vi "C_F.vi"() -> ()   [LabVIEW 2014]
panel:
  in  "STOP":bool
  in  "Temp Scale":bool
  out "Thermometer":dbl(slide) scale=0.0..100.0
  # "C\n\nF"
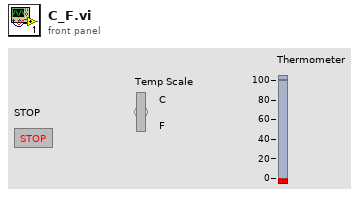
[diagram p1: front panel]
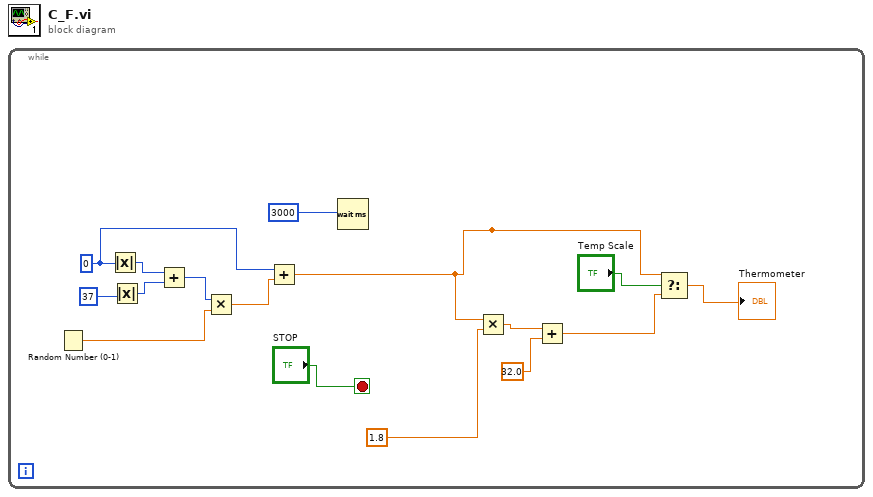
[diagram p0: block diagram]
diagram:
  n1 = while {
    stop <- "STOP" stop-if-true
    w11 = 0
    n2 = Random Number (0-1)() -> (number: 0 to 1=w13:dbl)
    n3 = Absolute Value(x=w11) -> (abs(x)=w15:i32)
    n4 = Absolute Value(x=37) -> (abs(x)=w14:i32)
    n5 = Add(x=w15, y=w14) -> (x+y=w12:i32)
    n6 = Multiply(x=w12, y=w13) -> (x*y=w10:dbl)
    n7 = Add(x=w11, y=w10) -> (x+y=w1:dbl)
    n8 = Wait (ms)(milliseconds to wait=3000) -> ()  [unwired: 1 out]
    n9 = Multiply(x=w1, y=1.8) -> (x*y=w4:dbl)
    n10 = Add(x=w4, y=32.0) -> (x+y=w7:dbl)
    n11 = Select(t=w1, s="Temp Scale", f=w7) -> (s? t:f=→"Thermometer":dbl)
  }
